vi "GT Compare Data.vi"(0 "cardNum":i16, 1 "encoder":i16, 2 "source":i16, 3 "pulseType":i16, 4 "startLevel":i16, 5 "time":i16, 6 "pBuf1":i32[](array[numeric]), 7 "error in (no error)":errorcluster caption="错误输入（无错误）", 8 "count1":i16, 10 "count2":i16, 11 "pBuf2":i32[](array[numeric])) -> (20 "function return":i16, 26 "pBuf1 out":i32[](array[numeric]), 27 "error out":errorcluster caption="错误输出")   [LabVIEW 2020, in "gts.lvlib"]
doc: "GT_API GT_CompareData(short cardNum,short encoder,short source,short pulseType,short startLevel,short time,\n long *pBuf1,short count1,long *pBuf2,short count2);"
uses:
  gts.lvlib
  dll/32bit/multi_card/gts.dll
panel:
  out "pBuf2 out":i32[](array[numeric])
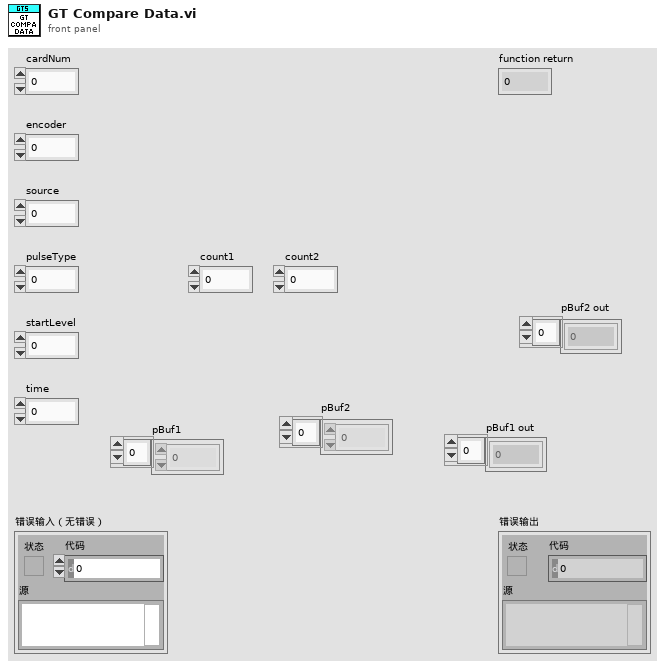
[diagram p1: front panel]
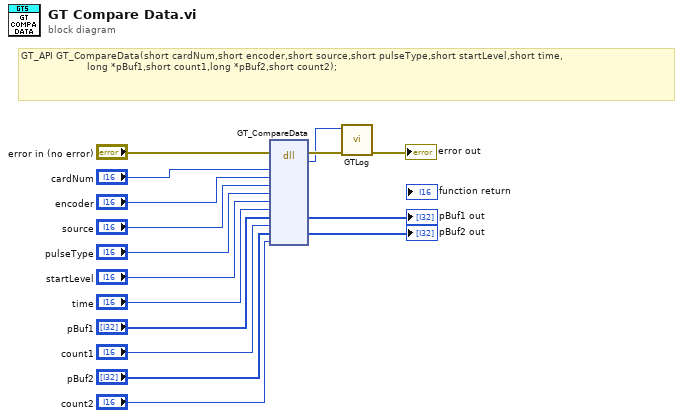
[diagram p0: block diagram]
diagram:
  # "GT_API GT_CompareData(short cardNum,short encoder,short source,short pulseType,short startLevel,short time,\n                      long *pBuf1,short count1,long *pBuf2,short count2);"
  n1 = dll-call lib="C:/1228/dll/32bit/multi_card/gts.dll" fn="GT_CompareData"(error in="error in (no error)", "cardNum"="cardNum", "encoder"="encoder", "source"="source", "pulseType"="pulseType", "startLevel"="startLevel", "time"="time", "pBuf1"="pBuf1", "count1"="count1", "pBuf2"="pBuf2", "count2"="count2") -> (error out=w6:errorcluster, "返回类型"=w1:i16, "pBuf1"=→"pBuf1 out":i32[], "pBuf2"=→"pBuf2 out":i32[])  [unwired: 10 in, 1 out]
  n2 = call "GTLog.vi"("error in (no error)"=w6, "Numeric"=w1) -> ("error out"=→"error out":errorcluster)  [unwired: 9 in]
